vi "Register Events to Controller.vi"(8 "error in (no error)":errorcluster, 11 "Example View in":refnum<class "Example View Actor 2.lvclass">) -> (0 "error out":errorcluster, 3 "Example View out":refnum<class "Example View Actor 2.lvclass">)   [LabVIEW 2023]
doc: "This dinamic dispatch methods has to be overriddent by the child sink classes to register events to the source"
uses:
  Event/Event.lvclass
  Example Events/Boolean Event.lvclass
  Example View Actor Messages/Example View Actor 2/Update Boolean Event Msg/Update Boolean Event Msg.lvclass
  View Actor/View Actor.lvclass
  C:/Projects/Shared Libraries/Event Actors/Event Data Types/Event Boolean/Event Boolean.lvclass
  C:/Projects/Shared Libraries/Event Actors/Event/Event.lvclass
  C:/Projects/Shared Libraries/Event Actors/Examples/Example Events/Boolean Event.lvclass
  C:/Projects/Shared Libraries/Event Actors/Event Handlers/Abstract Event Message for View/Abstract Event Message for View.lvclass
  C:/Program Files/National Instruments/LabVIEW 2023/vi.lib/ActorFramework/Message/Message.lvclass
  C:/Projects/Shared Libraries/Event Actors/Examples/Example View Actor/Example View Actor Messages/Example View Actor 2/Update Boolean Event Msg/Update Boolean Event Msg.lvclass
  Example View Actor 2.lvclass
  C:/Projects/Shared Libraries/Event Actors/View Actor/View Actor.lvclass
  C:/Program Files/National Instruments/LabVIEW 2023/vi.lib/ActorFramework/Actor/Actor.lvclass
  C:/Projects/Shared Libraries/Event Actors/Examples/Example View Actor/Example View Actor 2/Example View Actor 2.lvclass
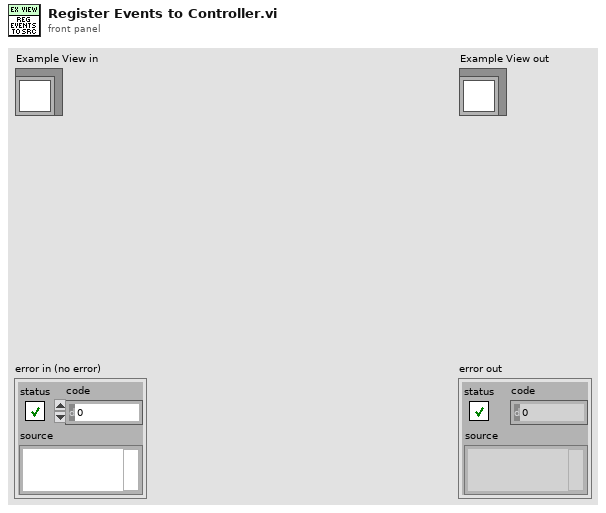
[diagram p1: front panel]
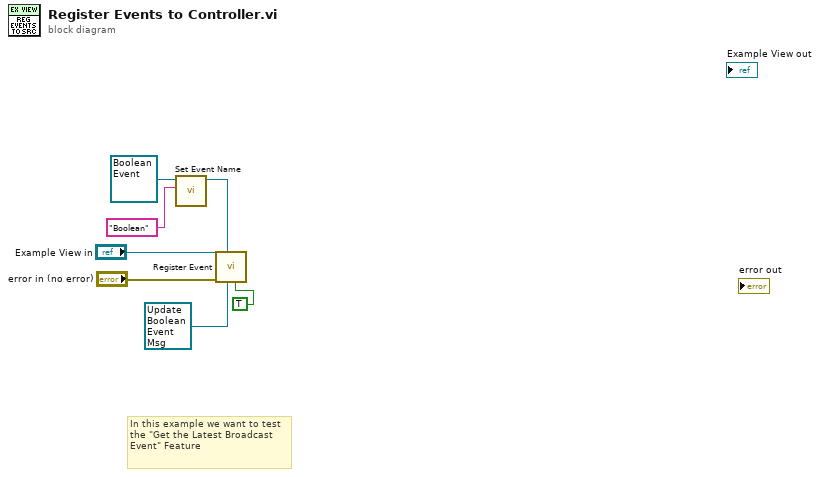
[diagram p0: block diagram]
diagram:
  # "In this example we want to test the \"Get the Latest Broadcast Event\" Feature"
  n1 = call "Set Event Name.vi"("Name (Generic)"="Boolean", "Event In"=refnum<class "Boolean Event.lvclass"> refnum ("Example Source.lvlib:Boolean Event.lvclass")) -> ("Event Out"=w2:refnum<class "Boolean Event.lvclass">)  [unwired: 9 in]
  n2 = call "Register Event.vi"("Get Last Broadcast Event (F)"=TRUE ("Get Last Broadcast Event (F)\""), "Event Handler"=refnum<class "Update Boolean Event Msg.lvclass"> refnum ("Update Time Msg.lvclass"), "Event"=w2, "error in (no error)"="error in (no error)", "View Actor in"="Example View in") -> ()  [unwired: 5 in, 2 out]
